vi "flip by cols.vi"(11 "Matrix":T1) -> (3 "Flipped by Cols":T1)   [LabVIEW 2019]
uses:
  <vilib>/Analysis/Matrix/Datatypes/RealMatrix.ctl
  <vilib>/Analysis/Matrix/Numeric/Conversions/Matrix To Array - RM.vi
  <vilib>/Analysis/Matrix/Numeric/Conversions/Array To Matrix - RA2.vi
  <vilib>/Analysis/Matrix/NI_Matrix.lvlib
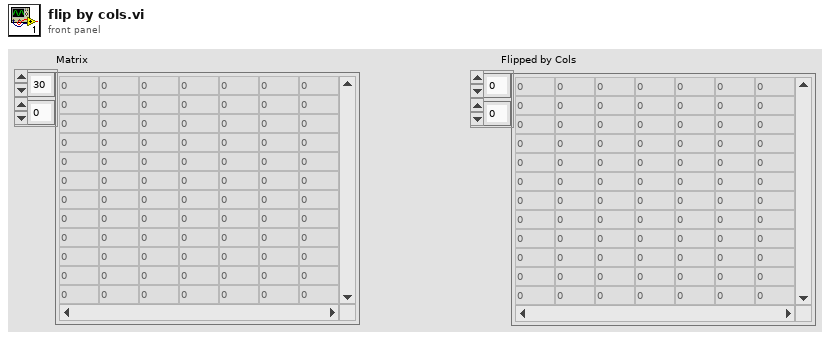
[diagram p1: front panel]
types:
  T1 = typedef "NI_Matrix.lvlib/RealMatrix.ctl" = dbl[][]
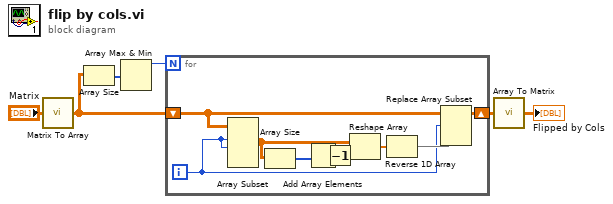
[diagram p0: block diagram]
diagram:
  n1 = call-poly <vilib>:"Matrix To Array.vi"("Real Matrix"="Matrix") -> ("Real 2D Array"=w5:dbl[][])
  n2 = Array Size(array=w5) -> (size(s)=w4:i32[])
  n3 = Array Max & Min(array=w4) -> (max value=w3:i32)  [unwired: 3 out]
  n4 = for {
    N: w3 -> [_]
    shift-right: [w9] -> w2
    shift-left: w5 -> [w14]
    i -> [w8]
    n5 = Array Subset(array=w14, index (row)=w8, length (row)=w8) -> (w11:dbl[][])  [unwired: 2 in]
    n6 = Array Size(array=w11) -> (size(s)=w13:i32[])
    n7 = Add Array Elements(numeric array=w13) -> (sum=w12:i32)
    n8 = Decrement(x=w12) -> (x-1=w7:i32)
    n9 = Reshape Array(w11, w7) -> (w10:dbl[])
    n10 = Reverse 1D Array(array=w10) -> (reversed array=w15:dbl[])
    n11 = Replace Array Subset(array=w14, new element=w15, index (row)=w8) -> (w9:dbl[][])  [unwired: 1 in]
  }
  n12 = call-poly <vilib>:"Array To Matrix.vi"("Real 2D Array"=w2) -> ("Real Matrix"=→"Flipped by Cols":T1)
